vi "Multi-Waveform Decimator.vi"(9 "Decimation #":i32=1 min=1, 10 "Old Y Values":dbl[][](array[numeric]), 11 "New Y Values":dbl[][](array[numeric])) -> (3 "Output Y Values":dbl[][](array[numeric]))   [LabVIEW 2014]
panel:
  # "Multi-Waveform Decimator"
  # "Inputs"
  # "Outputs"
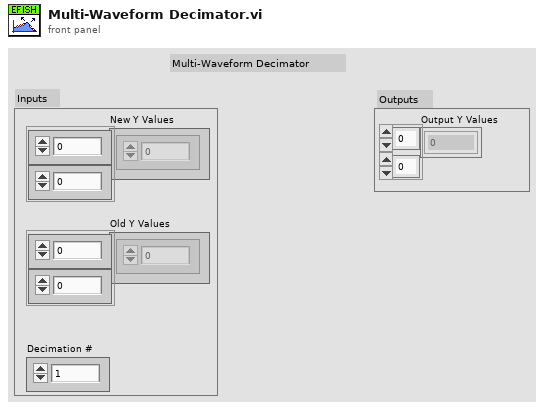
[diagram p1: front panel]
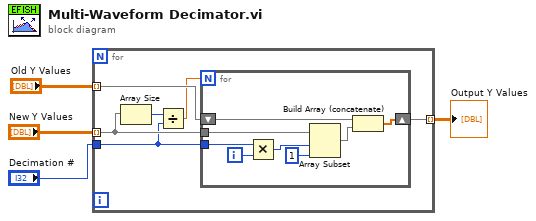
[diagram p0: block diagram]
diagram:
  n1 = for {
    tunnel: "New Y Values" -> [w7] mode=indexing
    tunnel: "Old Y Values" -> [w10] mode=indexing
    tunnel: "Decimation #" -> [w6]
    tunnel: [w5] -> w1 mode=indexing
    n2 = Array Size(array=w7) -> (size(s)=w9:i32)
    n3 = Divide(x=w9, y=w6) -> (x/y=w8:dbl)
    n4 = for {
      N: w8 -> [_]
      shift-right: [w11] -> w5
      shift-left: w10 -> [w13]
      tunnel: w7 -> [w16]
      tunnel: w6 -> [w18]
      i -> [w17]
      n5 = Multiply(x=w18, y=w17) -> (x*y=w15:i32)
      n6 = Array Subset(array=w16, index=w15, length=1) -> (w12:dbl[])
      n7 = Build Array (concatenate)(w13, w12) -> (w11:dbl[])
    }
  }
  "Output Y Values" <- w1
